vi "Read_queue_names.vi"(2 "error in (no error)":errorcluster, 3 "Queue in":refnum<queue>) -> (0 "error out":errorcluster, 1 "Array":string[](array[string]))   [LabVIEW 2017]
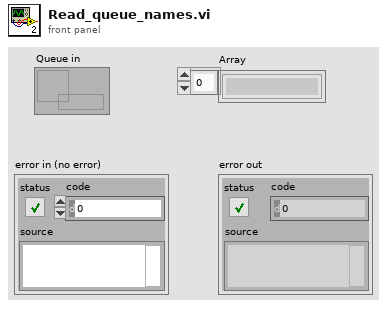
[diagram p1: front panel]
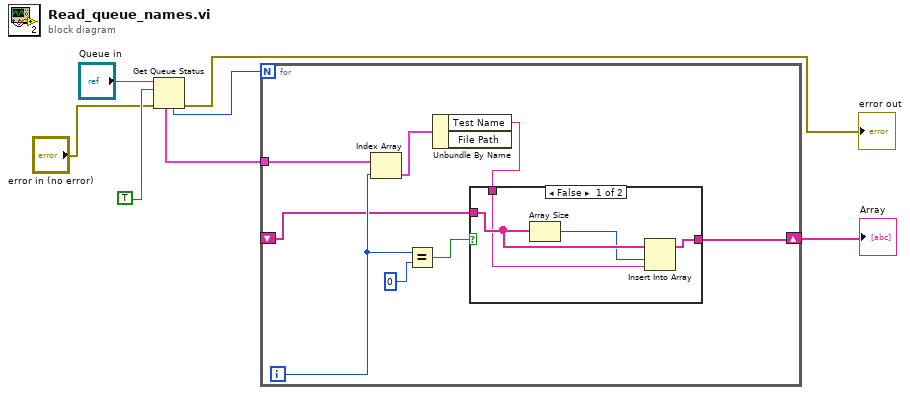
[diagram p0: block diagram]
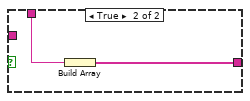
[diagram p2: hidden frame]
diagram:
  n1 = Get Queue Status(queue="Queue in", return elements? (F)=TRUE, error in (no error)="error in (no error)") -> (error out=→"error out":errorcluster, # elements in queue=w6:i32, elements=w5:cluster{"Test Name":string, "File Path":path}[])  [unwired: 5 out]
  n2 = for {
    N: w6 -> [_]
    tunnel: w5 -> [w15]
    shift-right: [w9] -> w4
    shift-left: _ -> [w8]
    i -> [w14]
    n3 = Index Array(array=w15, index=w14) -> (element=w11:cluster{"Test Name":string, "File Path":path})
    n4 = Equal?(x=w14, y=0) -> (x = y?=w12:bool)
    n5 = Unbundle By Name(w11) -> ("Test Name"=w10:string)  [unwired: 1 out]
    n6 = case shown="False" w12 {
      tunnel: w10 -> [w17 w21]
      tunnel: [w18 w20] -> w9
      tunnel: w8 -> [w19 _]
      frame False {
        n7 = Array Size(array=w19) -> (size(s)=w16:i32)
        n8 = Insert Into Array(array=w19, index=w16, new element=w17) -> (w18:string[])
      }
      frame True {
        n9 = Build Array(w21) -> (w20:string[])
      }
    }
  }
  "Array" <- w4
